vi "move_abs.vi"(8 "error in":errorcluster, 10 "Position Aboslute":i32, 11 "VISA in":refnum<visa-resource-name>) -> (0 "error out":errorcluster, 3 "VISA out":refnum<visa-resource-name>)   [LabVIEW 2019]
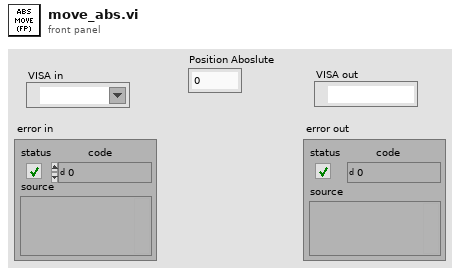
[diagram p1: front panel]
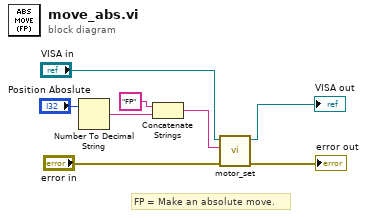
[diagram p0: block diagram]
diagram:
  # "FP = Make an absolute move."
  n1 = Number To Decimal String(number="Position Aboslute") -> (decimal integer string=w3:string)  [unwired: 1 in]
  n2 = Concatenate Strings("FP", w3) -> (w8:string)
  n3 = call "motor_set.vi"("error in"="error in", "command"=w8, "VISA in"="VISA in") -> ("error out"=→"error out":errorcluster, "VISA out"=→"VISA out":refnum<visa-resource-name>)  [unwired: 7 in]
